vi "Delete Subsystem.vi"(8 "error in (no error)":errorcluster, 10 "Subsystem":T1={"Name"="Control1", "Root URL"=""}, 11 "System Name":string) -> (0 "error out":errorcluster)   [LabVIEW 2024]
doc: "Deletes a subsystem in the shared variable engine."
uses:
  Controls/Server/Subsystem Configuration.ctl
  <vilib>/lvdsc/NI_DSC.lvlib
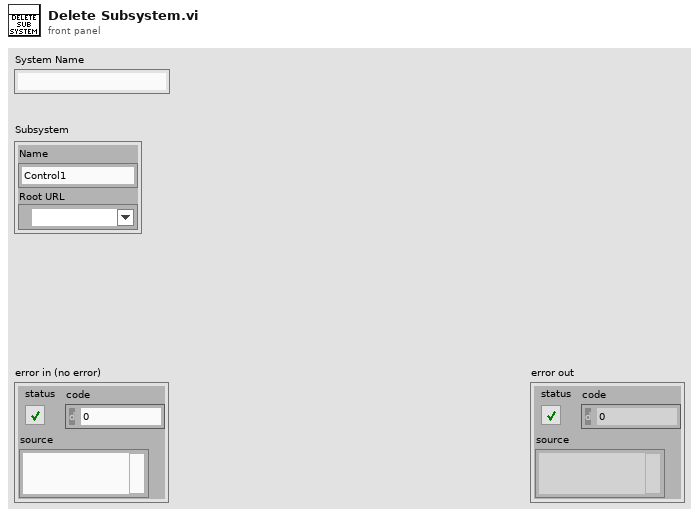
[diagram p1: front panel]
types:
  T1 = typedef "Subsystem Configuration.ctl" = cluster{"Name":string, "Root URL":refnum<k21>}
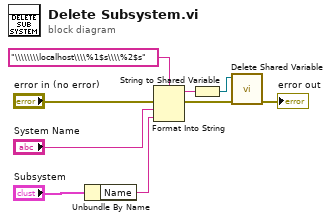
[diagram p0: block diagram]
diagram:
  n1 = Unbundle By Name("Subsystem") -> ("Name"=w2:string)
  n2 = Format Into String(format string="\\\\\\\\localhost\\\\%1$s\\\\%2$s", error in="error in (no error)", "System Name", w2) -> (resulting string=w6:string, error out=w4:errorcluster)  [unwired: 1 in]
  n3 = String to Shared Variable(0:w6) -> (2:w5:refnum<k21>)  [unwired: 1 out]
  n4 = call <vilib>:"Delete Shared Variable.vi"("error in (no error)"=w4, "shared variable"=w5) -> ("error out"=→"error out":errorcluster)  [unwired: 9 in]
